vi "week12_autoIt_automation_v10.vi"() -> ()   [LabVIEW 2010]
panel:
  in  "stop":bool
  in  "Time interval between running autoIt program":dbl=10.0
  in  "Link to COMPILED AutoIt program":path=path "autoit_example_LV-week3.exe"
  out "String":string="Step away from the mouse!"
  out "Progress until reset":dbl(slide) scale=0.0..10.0
  out "t0":dbl=451158247.0
  out "Elapsed time [sec]":dbl format="%.1f"
  out "end":dbl=10.0 format="%#_4g"
  # "seconds"
  # "0 sec"
  # "sec"
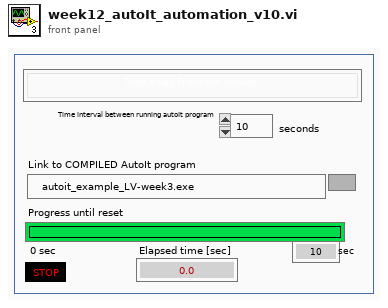
[diagram p1: front panel]
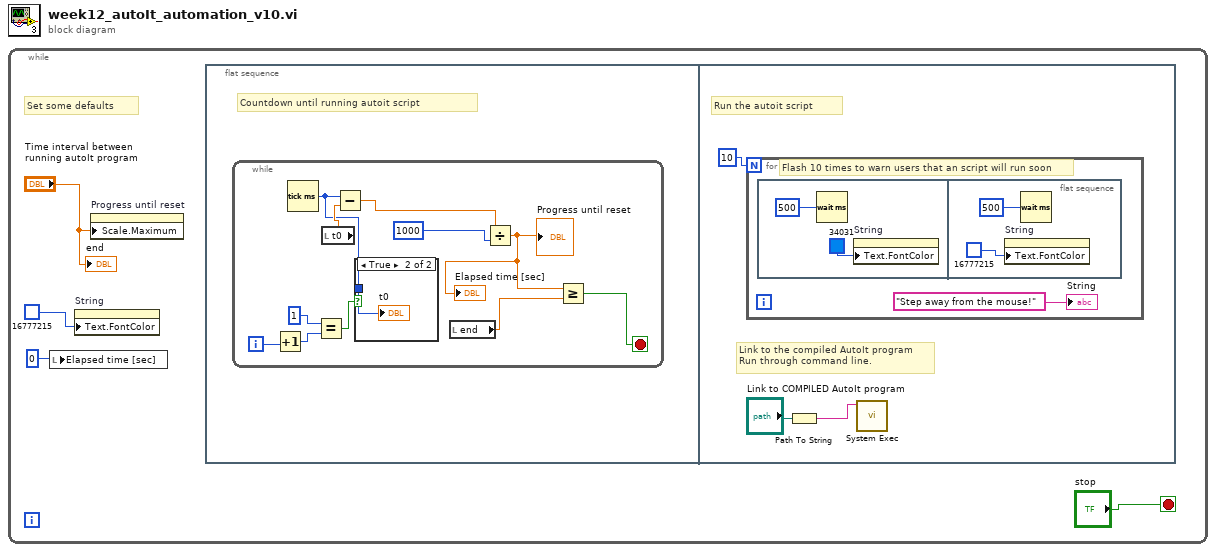
[diagram p0: block diagram]
diagram:
  n1 = while {
    stop <- "stop" stop-if-true
    # "Set some defaults"
    n2 = local write "Elapsed time [sec]"(0) -> ()
    n3 = property on="String" class="Str"("Text.FontColor"=u32 16777215) -> ()  [unwired: 2 in, 2 out]
    n4 = property on="Progress until reset" class="Slide (strict)"("Scale.Maximum"="Time interval between running autoIt program") -> ()  [unwired: 2 in, 2 out]
    n5 = flat-sequence {
      frame #0 {
        # "Countdown until running autoit script"
        n6 = while {
          i -> [w8]
          stop <- w9 stop-if-true
          n7 = Increment(x=w8) -> (x+1=w7:i32)
          n8 = Tick Count (ms)() -> (millisecond timer value=w13:u32)
          n9 = Equal?(x=1, y=w7) -> (x = y?=w12:bool)
          n10 = local read "t0"() -> (w14:dbl)
          n11 = Subtract(x=w13, y=w14) -> (x-y=w6:dbl)
          n12 = case shown="True" w12 {
            tunnel: w13 -> [_ w16]
            frame False {
            }
            frame True {
              "t0" <- w16
            }
          }
          n13 = local read "end"() -> (w10:dbl)
          n14 = Divide(x=w6, y=1000) -> (x/y=w15:dbl)
          "Elapsed time [sec]" <- w15
          "Progress until reset" <- w15
          n15 = Greater Or Equal?(x=w15, y=w10) -> (x >= y?=w9:bool)
        }
      }
      frame #1 {
        # "Run the autoit script"
        # "Link to the compiled AutoIt program\nRun through command line."
        n16 = for {
          N: 10 -> [_]
          # "Flash 10 times to warn users that an script will run soon"
          n17 = flat-sequence {
            frame #0 {
              n18 = Wait (ms)(milliseconds to wait=500) -> ()  [unwired: 1 out]
              n19 = property on="String" class="Str"("Text.FontColor"=u32 34031) -> ()  [unwired: 2 in, 2 out]
            }
            frame #1 {
              n20 = property on="String" class="Str"("Text.FontColor"=u32 16777215) -> ()  [unwired: 2 in, 2 out]
              n21 = Wait (ms)(milliseconds to wait=500) -> ()  [unwired: 1 out]
            }
          }
          "String" <- "Step away from the mouse!"
        }
        n22 = Path To String(path="Link to COMPILED AutoIt program") -> (string=w19:string)
        n23 = call <vilib>:"System Exec.vi"("command line"=w19) -> ()  [unwired: 7 in, 4 out]
      }
    }
    "end" <- "Time interval between running autoIt program"
  }
